vi "Global - All UI Loop Stop.vi"() -> ()   [LabVIEW 2020]
panel:
  in  "All UI Loop Stop":bool
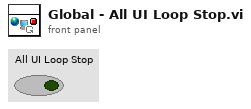
[diagram p1: front panel]
diagram:
